vi "Change Base Address Benchmark.vi"() -> ()   [LabVIEW 2016]
uses:
  <vilib>/Platform/TimedLoop/XDataNode/timing_clust.ctl
  <vilib>/Platform/TimedLoop/XDataNode/nitl_modes.ctl
  <vilib>/Platform/TimedLoop/XDataNode/wakeup.ctl
  Source/GE 5565PIORC/GE 5565PIORC.lvclass/GE 5565PIORC.ctl
  Source/GE 5565PIORC/VIs/Registers/Local Configuration.LAS1RR.Address Range.Get.vi
  Source/GE 5565PIORC/VIs/Registers/Local Configuration.Get Register Offset.vi
  Source/GE 5565PIORC/GE 5565PIORC.lvclass
  <vilib>/platform/TimedLoop/XDataNode/XDataNode.xnode
  <vilib>/Platform/TimedLoop/XDataNode/XDNodeRunTimeDep.lvlib
panel:
  out "Local Base Address":u32 format="%.0x"
  out "Duration":dbl
  in  "VISA resource name":refnum<visa-resource-name>
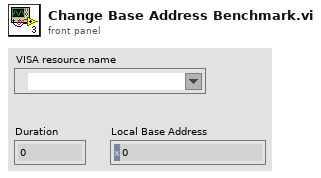
[diagram p1: front panel]
types:
  T1 = typedef "XDNodeRunTimeDep.lvlib/timing_clust.ctl" = cluster{"Expected End [f-1]":u64, "Actual End [f-1]":u64, "Finished Late? [f-1]":bool, "Expected End [i-1]":u64, "Actual End [i-1]":u64, "Finished Late? [i-1]":bool, "Expected Start [i]":u64, "Actual Start [i]":u64, "Expected Start [f]":u64, "Actual Start [f]":u64, "Source Name":string, "Structure Name":string, "Period":i64, "Deadline":i64, "Offset":i64, "Start":i64, "Priority":i32, "Timeout":i32, "Mode":T2, "Wakeup Reason":T3, "Error":errorcluster, "Source Type":string, "Secondary Source Type":string, "Global End Time":u64, "Global Start Time":u64, "Frame Duration":u64, "Iteration Duration":u64, "Assigned CPU":i32, "I/O Scan Engine Mode":u32}
  T2 = typedef "XDNodeRunTimeDep.lvlib/nitl_modes.ctl" = enum32{"No Change", "Process missed periods, maintain original phase", "Discard missed periods, maintain original phase", "Process missed periods, ignore original phase", "Discard missed periods, ignore original phase"}
  T3 = typedef "XDNodeRunTimeDep.lvlib/wakeup.ctl" = enum32{"Normal", "Aborted", "Asynchronous wakeup", "Timing source error", "Timed loop error", "Timeout"}
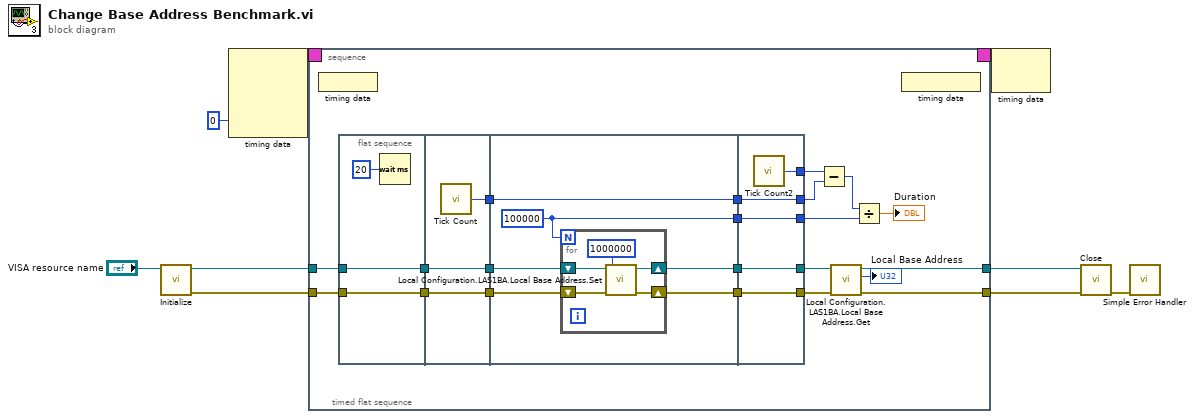
[diagram p0: block diagram]
diagram:
  n1 = call "Initialize.vi"("VISA resource name"="VISA resource name") -> ("error out"=w3:errorcluster, "GE 5565PIORC"=w4:refnum<class "GE 5565PIORC.lvclass">)  [unwired: 9 in]
  n2 = node-c288(0 ("Processor")) -> (w7:T1)  [unwired: 3 in]
  n3 = timed-sequence {
    timing: w7 -> [_]
    timing-out: [_] -> w6
    tunnel: w4 -> [w13]
    tunnel: w3 -> [w12]
    tunnel: [w11] -> w2
    tunnel: [w10] -> w1
    n4 = timed-flat-sequence {
      tunnel: w13 -> [w30]
      tunnel: w12 -> [w29]
      tunnel: [w16] -> w11
      tunnel: [w15] -> w10
      n5 = node-c288() -> ()  [unwired: 1 in]
      n6 = flat-sequence {
        tunnel: w30 -> [w36]
        tunnel: w29 -> [w35]
        tunnel: [w36] -> w27
        tunnel: [w35] -> w25
        tunnel: [w40] -> w34
        tunnel: [w39] -> w28
        tunnel: w27 -> [w39]
        tunnel: [w38] -> w26
        tunnel: w25 -> [w38]
        tunnel: w34 -> [w46]
        tunnel: [w46] -> w33
        tunnel: w28 -> [w45]
        tunnel: w26 -> [w44]
        tunnel: [w43] -> w24
        tunnel: [w42] -> w23
        tunnel: [w41] -> w22
        tunnel: [w56] -> w32
        tunnel: [w55] -> w31
        tunnel: w33 -> [w55]
        tunnel: w24 -> [w54]
        tunnel: w23 -> [w53]
        tunnel: [w54] -> w18
        tunnel: [w53] -> w17
        tunnel: w22 -> [w52]
        tunnel: [w52] -> w20
        frame #0 {
          n7 = Wait (ms)(milliseconds to wait=u32 20) -> ()  [unwired: 1 out]
        }
        frame #1 {
          n8 = call "Tick Count"() -> ("Tick Count(uSec)"=w40:u32)
        }
        frame #2 {
          w41 = 100000
          n9 = for {
            N: w41 -> [_]
            shift-right: [w49] -> w43
            shift-left: w45 -> [w51]
            shift-right: [w48] -> w42
            shift-left: w44 -> [w50]
            n10 = call "Local Configuration.LAS1BA.Local Base Address.Set.vi"("error in (no error)"=w50, "Local Base Address"=u32 1000000, "GE 5565PIORC"=w51) -> ("error out"=w48:errorcluster, "GE 5565PIORC out"=w49:refnum<class "GE 5565PIORC.lvclass">)  [unwired: 7 in]
          }
        }
        frame #3 {
          n11 = call "Tick Count2"() -> ("Tick Count(uSec)"=w56:u32)
        }
      }
      n12 = Subtract(x=w32, y=w31) -> (x-y=w21:u32)
      n13 = call "Local Configuration.LAS1BA.Local Base Address.Get.vi"("error in (no error)"=w17, "GE 5565PIORC"=w18) -> ("error out"=w15:errorcluster, "Local Base Address"=→"Local Base Address":u32, "GE 5565PIORC out"=w16:refnum<class "GE 5565PIORC.lvclass">)  [unwired: 7 in]
      n14 = Divide(x=w21, y=w20) -> (x/y=→"Duration":dbl)
      n15 = node-c288() -> ()  [unwired: 1 out]
    }
  }
  n16 = node-c288(w6) -> ()  [unwired: 1 out]
  n17 = call "Close.vi"("error in (no error)"=w1, "GE 5565PIORC in"=w2) -> ("error out"=w8:errorcluster)  [unwired: 8 in, 1 out]
  n18 = call <vilib>:"Simple Error Handler.vi"("error in (no error)"=w8) -> ()  [unwired: 4 in, 5 out]
